vi "DMLSFM_STROBE_SIMPLE.vi"() -> ()   [LabVIEW 2017]
doc: "This example demonstrates how to generate a finite amount of digital data based off of a sample clock.\n\nSome hardware (e.g. M Series DAQ) must use an external sample clock for digital tasks. To view a complete list of available sample clock sources, consult the Device Routes table in Measurement and Automation Explorer.\n\nFor instructions on how to connect your signals to the DAQ device, refer to your device documentation."
uses:
  <vilib>/Utility/error.llb/DialogType.ctl
  <vilib>/DAQmx/write.llb/DAQmx Write (Analog 2D DBL NChan NSamp).vi
  <vilib>/DAQmx/create/channels.llb/DAQmx Create Channel (AO-Voltage-Basic).vi
  <vilib>/DAQmx/configure/timing.llb/DAQmx Timing (Sample Clock).vi
  <vilib>/DAQmx/configure/trigger.llb/DAQmx Start Trigger (Digital Edge).vi
  <vilib>/DAQmx/miscellaneous.llb/DAQmx Fill In Error Info.vi
  <resource>/objmgr/daqmx.rc
panel:
  out "error out":errorcluster
  in  "Start.Retriggerable":bool=TRUE
  in  "Digital Trigger Source":tag="/Dev4/PFI1"
  in  "Edge":i32(ring)=10280 items=["Rising"=10280, "Falling"=10171]
  in  "stop":bool
  in  "Sample Clock Source":tag="OnboardClock"
  out "Actual Sample Rate":dbl=1972.3865877712033 format="%0.2f"
  in  "Line(s)":tag="Dev4/ao0:1"
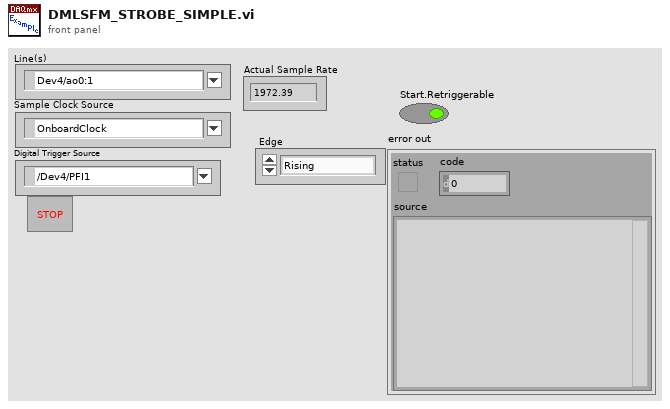
[diagram p1: front panel]
types:
  T1 = typedef "DialogType.ctl" = u16
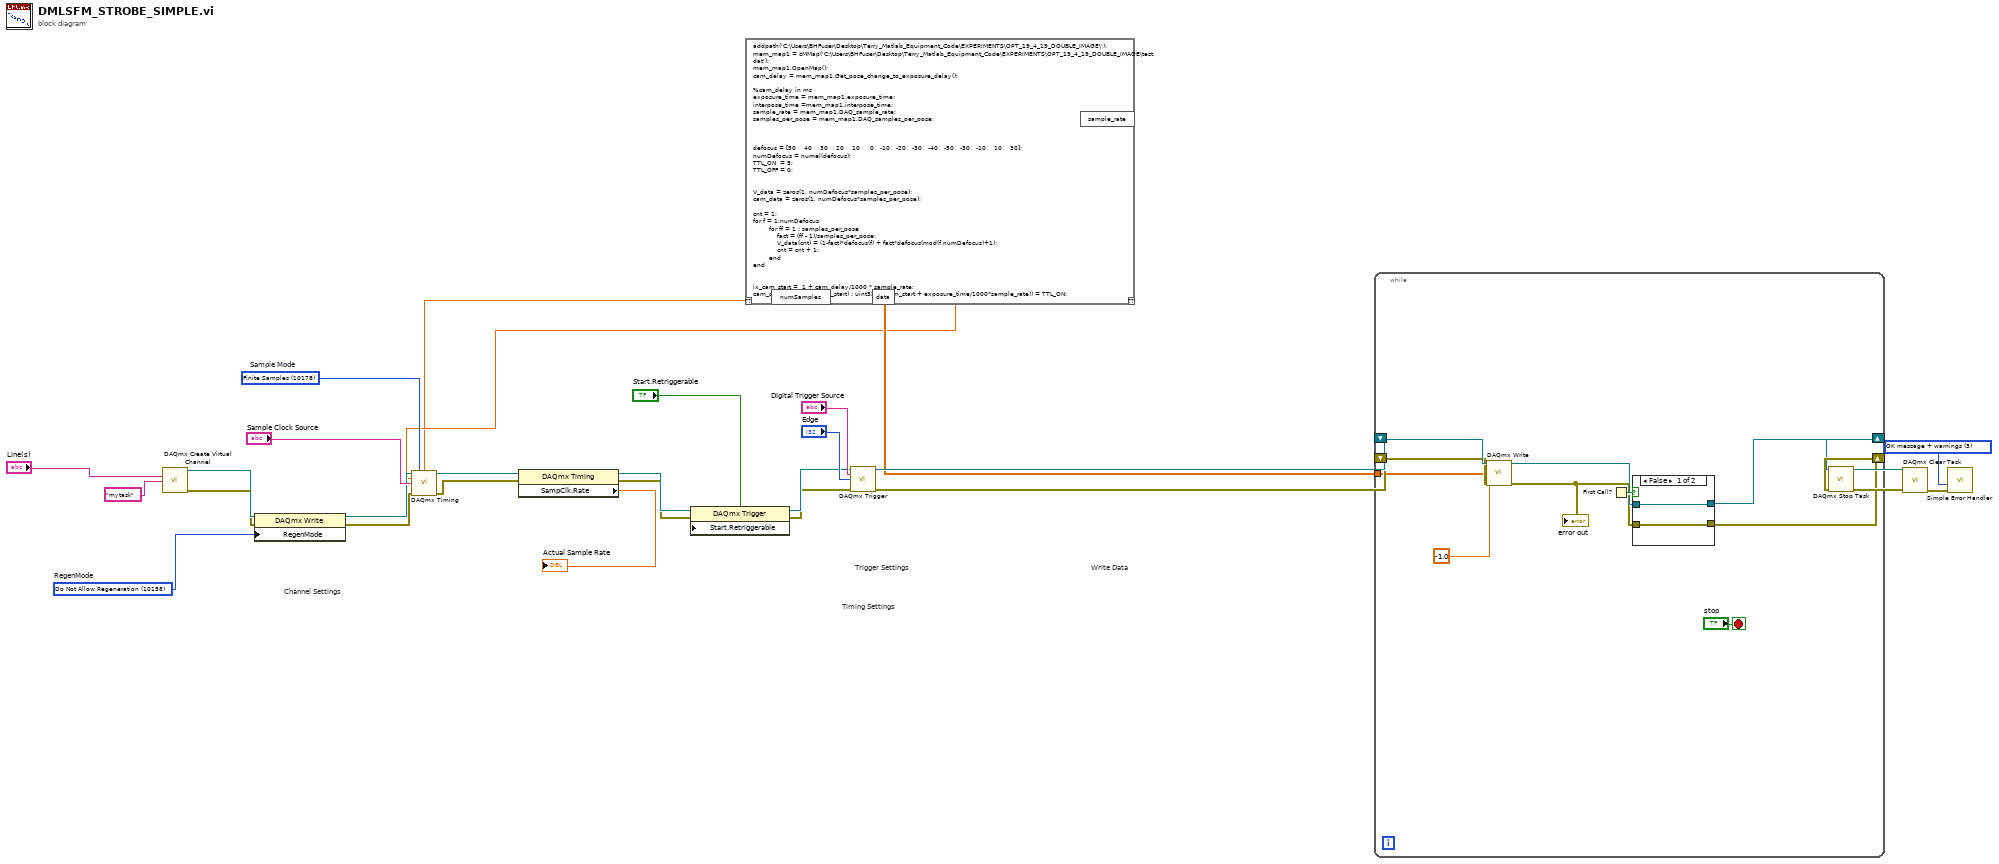
[diagram p0: block diagram]
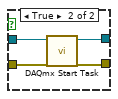
[diagram p2: hidden frame]
diagram:
  w7 = 10158 items=["Allow Regeneration"=10097, "Do Not Allow Regeneration"=10158]  # RegenMode
  w24 = T1 3 items=["no dialog", "OK message", "continue or stop message", "OK message + warnings", "continue/stop + warnings"] ("type of dialog (OK msg:1)")
  w25 = 10178 items=["Finite Samples"=10178, "Continuous Samples"=10123, "Hardware Timed Single Point"=12522]  # Sample Mode
  # "Trigger Settings"
  # "Timing Settings"
  # "Write Data"
  # "Channel Settings"
  n1 = call-poly <vilib>:"DAQmx Create Virtual Channel.vi"("physical channels"="Line(s)", "name to assign"="mytask") -> ("task out"=w11:refnum<k21>, "error out"=w9:errorcluster)  [unwired: 12 in]
  n2 = property class="DAQmx Write"(reference=w11, error in=w9, "RegenMode"=w7) -> (reference out=w10:refnum<k21>, error out=w8:errorcluster)
  n3 = script code="addpath('C:\\Users\\BHFuser\\Desktop\\Terry_Matlab_Equipment_Code\\EXPERIMENTS\\OPT_19_4_19_DOUBLE_IMAGE\\');\nmem_map1 = cMMap('C:\\Users\\BHFuser\\Desktop\\Terry_Matlab_Equipment_Code\\EXPERIMENTS\\OPT_19_4_19_DOUBLE_IMAGE\\test.dat');\nmem_map1.OpenMap(); \ncam_delay = mem_map1.Get_pose_change_to_exposure_delay();\n\n%cam_delay in ms\nexposure_time = mem_map1.exposure_time;\ninterpose_time =mem_map1.interpose_time;\nsample_rate = mem_map1.DAQ_sample_rate;\nsamples_per_pose = mem_map1.DAQ_samples_per_pose;\n\n\n\ndefocus = [50    40    30    20    10     0   -10   -20   -30   -40   -50   -30   -10    10    30];\nnumDefocus = numel(defocus);\nTTL_ON  = 5;\nTTL_OFF = 0;\n\n\nV_data = zeros(1, numDefocus*samples_per_pose);\ncam_data = zeros(1, numDefocus*samples_per_pose);\n\ncnt = 1;\nfor f = 1:numDefocus\n        for ff = 1 : samples_per_pose\n            fact = (ff - 1)/samples_per_pose;\n            V_data(cnt) = (1-fact)*defocus(f) + fact*defocus(mod(f,numDefocus)+1);\n            cnt = cnt + 1;\n        end\nend\n\n\nix_cam_start =  1 + cam_delay/1000 * sample_rate;\ncam_data( uint32(ix_cam_start) : uint32(ix_cam_start + exposure_time/1000*sample_rate)) = TTL_ON;\n\n        \n       \nnumSamples = numel(V_data);\nV_data = 0.271 - 0.00173 * V_data - 0.0000017*V_data.^2;\ndata = double([cam_data; V_data]);"() -> ("data"=w3:dbl[][], "sample_rate"=w2:dbl, "numSamples"=w1:dbl)  [unwired: 1 in, 1 out]
  n4 = call-poly <vilib>:"DAQmx Timing.vi"("task/channels in"=w10, "sample mode"=w25, "samples per channel"=w1, "rate"=w2, "source"="Sample Clock Source", "error in"=w8) -> ("task out"=w27:refnum<k21>, "error out"=w12:errorcluster)  [unwired: 8 in]
  n5 = property class="DAQmx Timing"(reference=w27, error in=w12) -> (reference out=w20:refnum<k21>, error out=w19:errorcluster, "SampClk.Rate"=→"Actual Sample Rate":dbl)
  n6 = property class="DAQmx Trigger"(reference=w20, error in=w19, "Start.Retriggerable"="Start.Retriggerable") -> (reference out=w18:refnum<k21>, error out=w17:errorcluster)
  n7 = call-poly <vilib>:"DAQmx Trigger.vi"("task/channels in"=w18, "source"="Digital Trigger Source", "edge"="Edge", "error in"=w17) -> ("task out"=w5:refnum<k21>, "error out"=w4:errorcluster)  [unwired: 10 in]
  n8 = while {
    shift-right: [w38] -> w13
    shift-left: w4 -> [w34]
    shift-right: [w37] -> w6
    shift-left: w5 -> [w36]
    tunnel: w3 -> [w31]
    stop <- "stop" stop-if-true
    n9 = call-poly <vilib>:"DAQmx Write.vi"("task/channels in"=w36, "data"=w31, "timeout"=-1.0, "error in"=w34) -> ("task out"=w35:refnum<k21>, "error out"=w33:errorcluster)  [unwired: 9 in, 1 out]
    "error out" <- w33
    n10 = First Call?() -> (First Call?: T/F=w39:bool)
    n11 = case shown="False" w39 {
      tunnel: w35 -> [w41 w46]
      tunnel: w33 -> [w42 w45]
      tunnel: [w41 w44] -> w37
      tunnel: [w42 w43] -> w38
      frame False {
      }
      frame True {
        n12 = call <vilib>:"DAQmx Start Task.vi"("task/channels in"=w46, "error in"=w45) -> ("task out"=w44:refnum<k21>, "error out"=w43:errorcluster)  [unwired: 12 in]
      }
    }
  }
  n13 = call <vilib>:"DAQmx Stop Task.vi"("task/channels in"=w6, "error in"=w13) -> ("task out"=w15:refnum<k21>, "error out"=w14:errorcluster)  [unwired: 12 in]
  n14 = call <vilib>:"DAQmx Clear Task.vi"("task in"=w15, "error in"=w14) -> ("error out"=w30:errorcluster)  [unwired: 13 in]
  n15 = call <vilib>:"Simple Error Handler.vi"("type of dialog (OK msg:1)"=w24, "error in (no error)"=w30) -> ()  [unwired: 3 in, 5 out]
